vi "Config.vi"(8 "error in (no error)":errorcluster, 10 "Setting":variant, 11 "Sim DC Power in":refnum<class "Sim DC Power.lvclass">) -> (0 "error out":errorcluster, 3 "Sim DC Power out":refnum<class "Sim DC Power.lvclass">)   [LabVIEW 2025, in "Power Supply.lvlib" / "Sim DC Power.lvclass"]
uses:
  Sim DC Power.lvclass
  Sim DC Power.lvclass/Sim DC Power.ctl
  PS Channel/Power Supply Channel.lvclass
  PS Channel configuration/Power Supply Channel configuration.lvclass
  Users/Public/Documents/Sandia National Labs/TSS Plugin/Abstract Engine.lvlibp/Plugin/Abstract/Abstract Instrument/Channel.ctl
  Users/Public/Documents/Sandia National Labs/TSS Plugin/Abstract Engine.lvlibp/Plugin/Abstract/Abstract Instrument/Abstract Instrument.lvclass
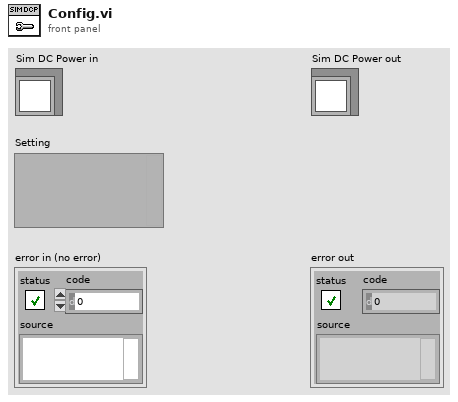
[diagram p1: front panel]
types:
  T1 = typedef "Abstract Engine.lvlibp/Abstract Instrument.lvclass/Channel.ctl" = cluster{"Alias":string, "DataType":enum16{"Anaolg Input", "Waveform"}, "Unit":enum16{"---", "V", "A", "Ohm", "Hz", "uF", "degC", "deg"}, "Upper limit":dbl, "Lower limit":dbl, "Measurement":variant}
  T2 = typedef "Power Supply.lvlib/Power Supply Channel configuration.lvclass/PS Channel Setting.ctl" = cluster{"Driver":string, "Pin":string, "Test Voltage":string, "Voltage Low":dbl, "Voltage Norminal":dbl, "Voltage High":dbl, "PreTest Voltage":dbl, "PreTest Current":dbl, "Current Limit":dbl}
  T3 = typedef "Abstract Engine.lvlibp/Channel configuration.lvclass/Default Channel.ctl" = cluster{"Address":string, "SW Alias":string, "Enabled":bool, "Type":string, "Description":string}
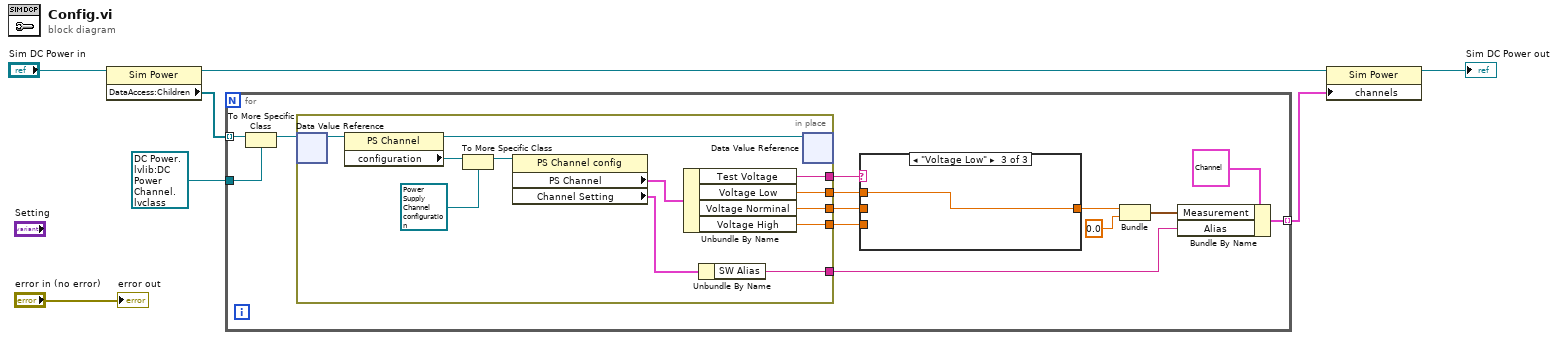
[diagram p0: block diagram]
diagram:
  n1 = property class="Sim Power"(reference="Sim DC Power in") -> (reference out=w5:refnum<class "Sim DC Power.lvclass">, "DataAccess:Children"=w4:refnum<data-value>[])  [unwired: 1 in, 1 out]
  n2 = for {
    tunnel: w4 -> [w19] mode=indexing
    tunnel: refnum<data-value> refnum ("data value reference") -> [w18]
    tunnel: [w13] -> w1 mode=indexing
    n3 = To More Specific Class(target class=w18, reference=w19) -> (specific class reference=w20:refnum<data-value>)  [unwired: 1 in, 1 out]
    n4 = in-place {
      in-place-border: [w28] -> w17
      in-place-border: [w27] -> w16
      in-place-border: [w26] -> w15
      in-place-border: [w25] -> w14
      in-place-border: [w24] -> w12
      # "Initialize the front panel controls when loaded"
      n5 = in-place-dvr #1(w20) -> (w35:refnum<class "Power Supply Channel.lvclass">)  [unwired: 1 out]
      n6 = property class="PS Channel"(reference=w35) -> (reference out=w34:refnum<class "Power Supply Channel.lvclass">, "configuration"=w33:refnum<class "CEF_serializable configuration.lvclass">)  [unwired: 1 in, 1 out]
      n7 = To More Specific Class(target class=refnum<class "Power Supply Channel configuration.lvclass"> refnum ("DC Power.lvlib:DCPower Channel configuration.lvclass"), reference=w33) -> (specific class reference=w31:refnum<class "Power Supply Channel configuration.lvclass">)  [unwired: 1 in, 1 out]
      n8 = property class="PS Channel config"(reference=w31) -> ("PS Channel"=w30:T2, "Channel Setting"=w29:T3)  [unwired: 1 in, 2 out]
      n9 = Unbundle By Name(w30) -> ("Test Voltage"=w28:string, "Voltage Low"=w27:dbl, "Voltage Norminal"=w26:dbl, "Voltage High"=w25:dbl)
      n10 = Unbundle By Name(w29) -> ("SW Alias"=w24:string)
      n11 = in-place-dvr #1(w34) -> ()  [unwired: 2 out]
    }
    n12 = case shown="\"Voltage Low\"" w17 {
      tunnel: w16 -> [_ _ w23]
      tunnel: w15 -> [w21 _ _]
      tunnel: w14 -> [_ w22 _]
      tunnel: [w21 w22 w23] -> w11
      frame "Voltage Norminal", Default {
      }
      frame "Voltage High" {
      }
      frame "Voltage Low" {
      }
    }
    n13 = Bundle("Voltage Low"=w11, "Voltage Low"=0.0) -> (w9:cluster{"Voltage Low":dbl, "Voltage Low":dbl})  [unwired: 1 in]
    n14 = Bundle By Name(cluster=T1 {"Alias"="ch0", "DataType"=enum."Anaolg Input", "Unit"=enum."V", "Upper limit"=10.0, "Lower limit"=-10.0, "Measurement"=variant} ("Channel"), "Measurement"=w9, "Alias"=w12) -> (w13:T1)
  }
  n15 = property class="Sim Power"(reference=w5, "channels"=w1) -> (reference out=→"Sim DC Power out":refnum<class "Sim DC Power.lvclass">)  [unwired: 1 in, 1 out]
  "error out" <- "error in (no error)"
